vi "Read Alicat Type.vi"(8 "error in":errorcluster, 11 "Alicat Data in":refnum<class "Alicat Data.lvclass">) -> (0 "error out":errorcluster, 2 "Type":string, 3 "Alicat Data out":refnum<class "Alicat Data.lvclass">)   [LabVIEW 2014, in "Alicat Lib.lvlib" / "Alicat Data.lvclass"]
uses:
  Alicat Data.lvclass
  Alicat Data.lvclass/Alicat Data.ctl
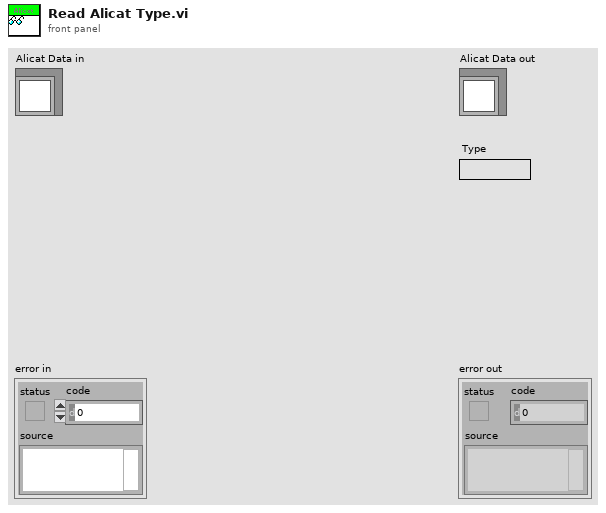
[diagram p1: front panel]
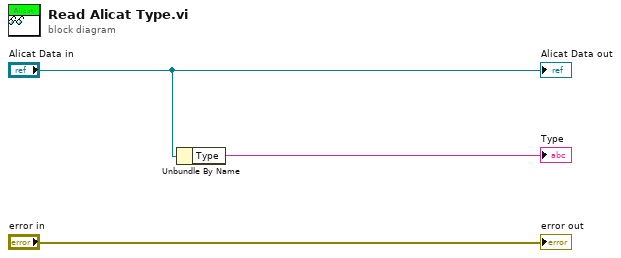
[diagram p0: block diagram]
diagram:
  n1 = Unbundle By Name("Alicat Data in") -> ("Type"=→"Type":string)
  "error out" <- "error in"
  "Alicat Data out" <- "Alicat Data in"
